vi "mqttBrokerWrite.vi"(0 "mqtt in":refnum<class "mqtt.lvclass">, 5 "broker":T1, 11 "error in (no error)":errorcluster) -> (4 "mqtt out":refnum<class "mqtt.lvclass">, 15 "error out":errorcluster)   [LabVIEW 2021, in "mqtt.lvclass"]
uses:
  mqtt.lvclass
  mqttTypedef/mqttBroker.ctl
  mqtt.lvclass/mqtt.ctl
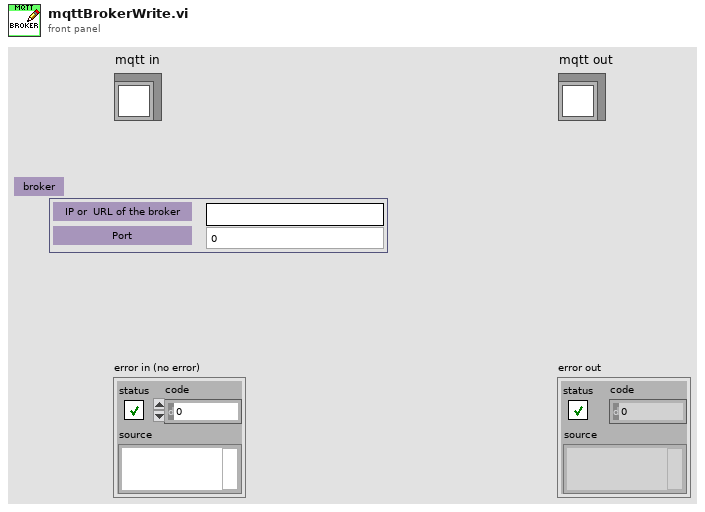
[diagram p1: front panel]
types:
  T1 = typedef "mqttBroker.ctl" = cluster{"IP or  URL of the broker":string, "connTimeout":i32, "writeTimeout":i32, "readTimeout":i32, "subTimeout":i32, "Port":u16}
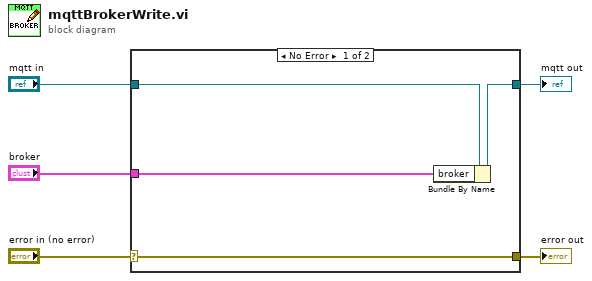
[diagram p0: block diagram]
diagram:
  n1 = case shown="No Error" "error in (no error)" {
    selector: "error in (no error)" -> [w9 w10]
    tunnel: [w9 w10] -> w4
    tunnel: [w8 w11] -> w2
    tunnel: "mqtt in" -> [w6 w11]
    tunnel: "broker" -> [w7 _]
    frame No Error {
      n2 = Bundle By Name(cluster=w6, "broker"=w7) -> (w8:refnum<class "mqtt.lvclass">)
    }
    frame Error {
    }
  }
  "error out" <- w4
  "mqtt out" <- w2
